vi "tank-overflow-detector.vi"() -> ()   [LabVIEW 2025]
panel:
  out "Slide 3":u8(slide) scale=0.0..10.0
  out "Slide 2":u8(slide) scale=0.0..10.0
  out "Slide":u8(slide) scale=0.0..10.0
  out "Tank 2":dbl(slide) scale=0.0..10.0
  out "Tank":dbl(slide) scale=0.0..10.0
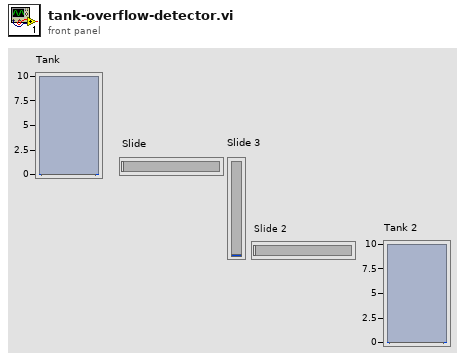
[diagram p1: front panel]
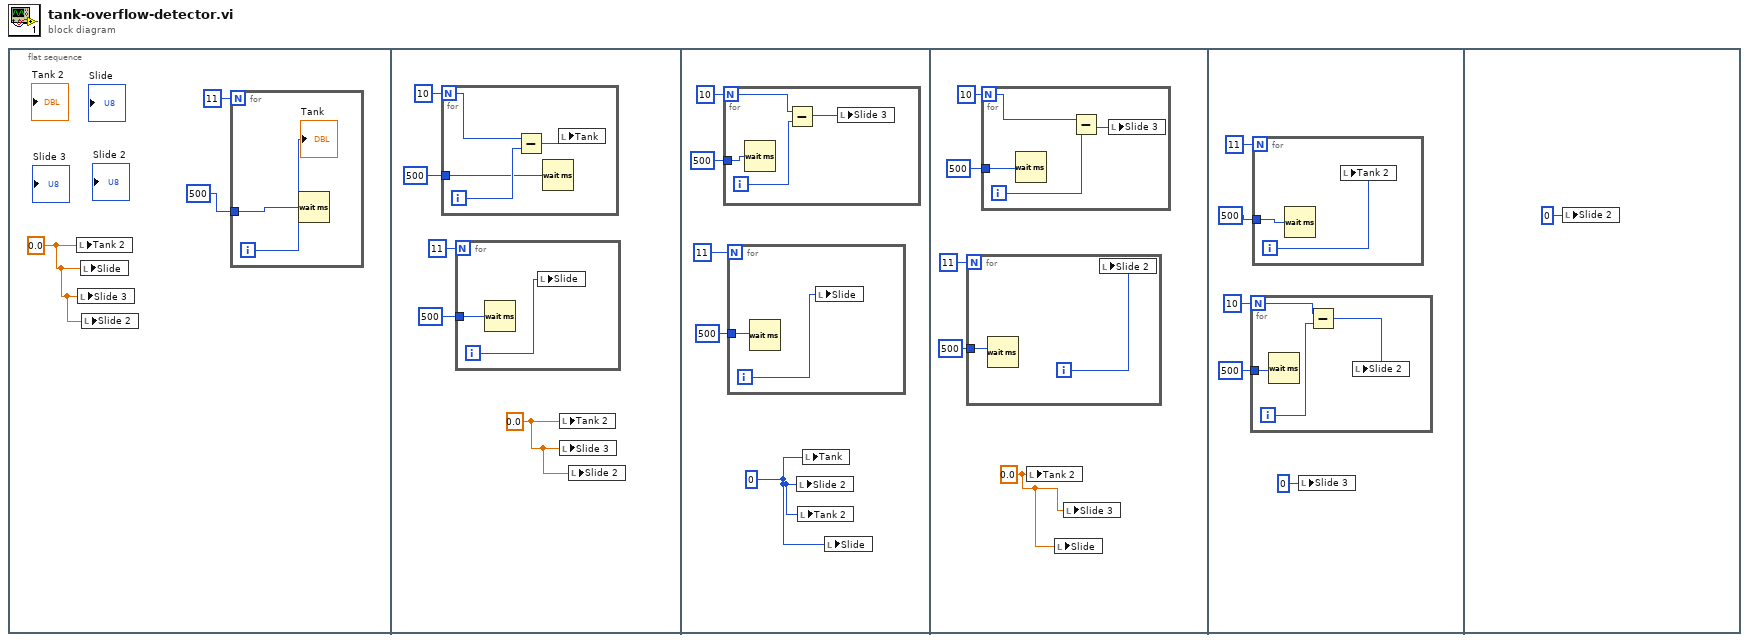
[diagram p0: block diagram]
diagram:
  n1 = flat-sequence {
    frame #0 {
      w3 = 0.0 ("Tank 2")
      n2 = local write "Tank 2"(w3) -> ()
      n3 = local write "Slide 3"(w3) -> ()
      n4 = local write "Slide"(w3) -> ()
      n5 = local write "Slide 2"(w3) -> ()
      n6 = for {
        N: 11 -> [_]
        tunnel: u32 500 ("milliseconds to wait") -> [w5]
        i -> [w4]
        n7 = Wait (ms)(milliseconds to wait=w5) -> ()  [unwired: 1 out]
        "Tank" <- w4
      }
    }
    frame #1 {
      w6 = 0.0 ("Tank 2")
      n8 = for {
        N: 10 -> [w15]
        tunnel: u32 500 ("milliseconds to wait") -> [w13]
        i -> [w16]
        n9 = Subtract(x=w15, y=w16) -> (x-y=w14:i32)
        n10 = Wait (ms)(milliseconds to wait=w13) -> ()  [unwired: 1 out]
        n11 = local write "Tank"(w14) -> ()
      }
      n12 = for {
        N: 11 -> [_]
        tunnel: u32 500 ("milliseconds to wait") -> [w11]
        i -> [w12]
        n13 = Wait (ms)(milliseconds to wait=w11) -> ()  [unwired: 1 out]
        n14 = local write "Slide"(w12) -> ()
      }
      n15 = local write "Tank 2"(w6) -> ()
      n16 = local write "Slide 3"(w6) -> ()
      n17 = local write "Slide 2"(w6) -> ()
    }
    frame #2 {
      w17 = u8 0 ("Slide 2")
      n18 = for {
        N: 10 -> [w26]
        tunnel: u32 500 ("milliseconds to wait") -> [w27]
        i -> [w25]
        n19 = Wait (ms)(milliseconds to wait=w27) -> ()  [unwired: 1 out]
        n20 = Subtract(x=w26, y=w25) -> (x-y=w24:i32)
        n21 = local write "Slide 3"(w24) -> ()
      }
      n22 = for {
        N: 11 -> [_]
        tunnel: u32 500 ("milliseconds to wait") -> [w23]
        i -> [w22]
        n23 = Wait (ms)(milliseconds to wait=w23) -> ()  [unwired: 1 out]
        n24 = local write "Slide"(w22) -> ()
      }
      n25 = local write "Slide 2"(w17) -> ()
      n26 = local write "Tank 2"(w17) -> ()
      n27 = local write "Tank"(w17) -> ()
      n28 = local write "Slide"(w17) -> ()
    }
    frame #3 {
      w28 = 0.0 ("Tank 2")
      n29 = for {
        N: 11 -> [_]
        tunnel: u32 500 ("milliseconds to wait") -> [w34]
        i -> [w33]
        n30 = Wait (ms)(milliseconds to wait=w34) -> ()  [unwired: 1 out]
        n31 = local write "Slide 2"(w33) -> ()
      }
      n32 = for {
        N: 10 -> [w37]
        tunnel: u32 500 ("milliseconds to wait") -> [w38]
        i -> [w36]
        n33 = Wait (ms)(milliseconds to wait=w38) -> ()  [unwired: 1 out]
        n34 = Subtract(x=w37, y=w36) -> (x-y=w35:i32)
        n35 = local write "Slide 3"(w35) -> ()
      }
      n36 = local write "Tank 2"(w28) -> ()
      n37 = local write "Slide"(w28) -> ()
      n38 = local write "Slide 3"(w28) -> ()
    }
    frame #4 {
      n39 = for {
        N: 10 -> [w44]
        tunnel: u32 500 ("millisecond timer value") -> [w47]
        i -> [w45]
        n40 = Wait (ms)(milliseconds to wait=w47) -> ()  [unwired: 1 out]
        n41 = Subtract(x=w44, y=w45) -> (x-y=w46:i32)
        n42 = local write "Slide 2"(w46) -> ()
      }
      n43 = for {
        N: 11 -> [_]
        tunnel: u32 500 ("milliseconds to wait") -> [w49]
        i -> [w48]
        n44 = Wait (ms)(milliseconds to wait=w49) -> ()  [unwired: 1 out]
        n45 = local write "Tank 2"(w48) -> ()
      }
      n46 = local write "Slide 3"(u8 0 ("Slide 3")) -> ()
    }
    frame #5 {
      n47 = local write "Slide 2"(u8 0 ("Slide 3")) -> ()
    }
  }
